vi "String functions.vi"() -> ()   [LabVIEW 2020]
panel:
  out "current time":timestamp
  out "String 6":string
  out "Boolean 2":bool
  out "Numeric 2":dbl
  out "Output Cluster":T1
  in  "String 5":string
  in  "Boolean":bool
  in  "Numeric":dbl
  out "replaced substring":string
  out "result string":string
  in  "length (len. of substring)":i32
  in  "offset (0) 2":i32
  in  "Substring":string
  in  "Main String":string
  out "substring":string
  in  "Input String":string
  in  "length (rest)":i32
  in  "offset (0)":i32
  out "concatenated string":string
  in  "String 4":string
  in  "String 3":string
  in  "String 2":string
  in  "String":string
  out "String Length":dbl
  in  "String Input":string
  # "(1)"
  # "(2)"
  # "(3)"
  # "(4)"
  # "(5)"
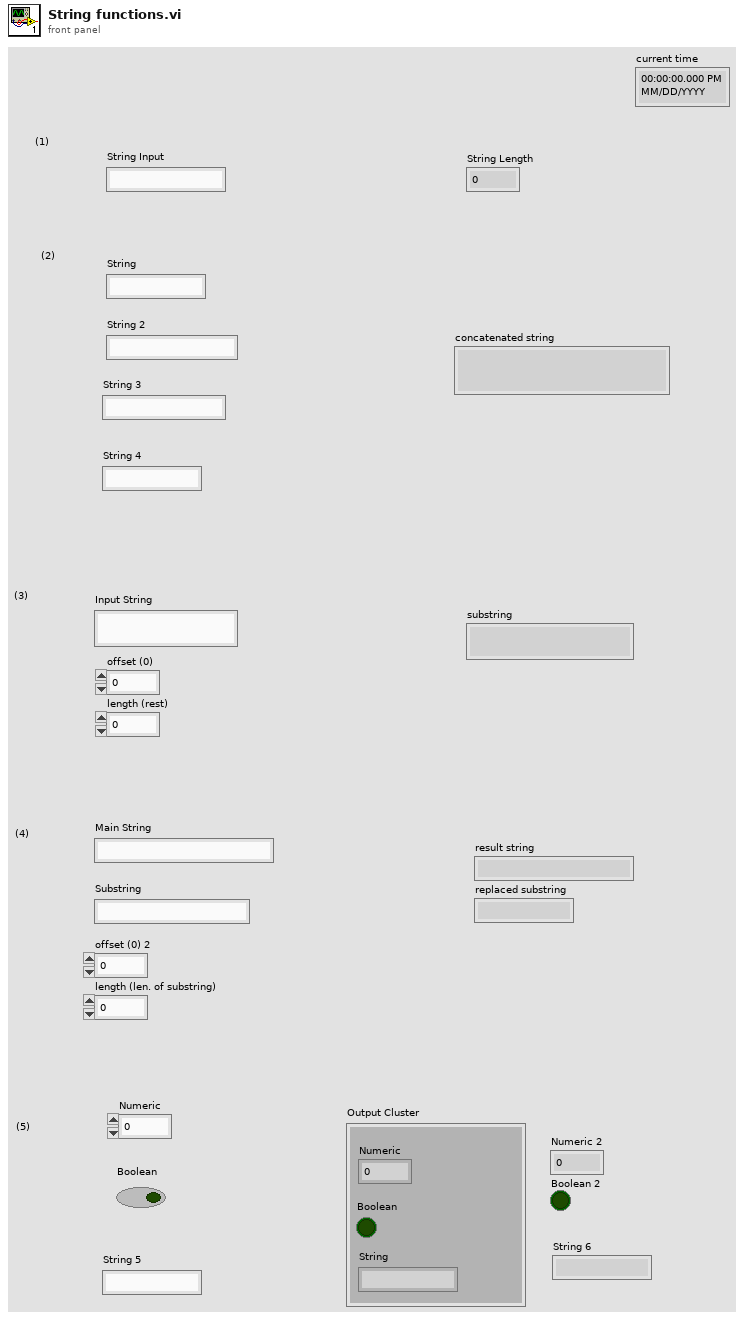
[diagram p1: front panel]
types:
  T1 = cluster{"Numeric":dbl, "Boolean":bool, "String":string}
  T2 = cluster{"Numeric":dbl, "Boolean":bool, "String 5":string}
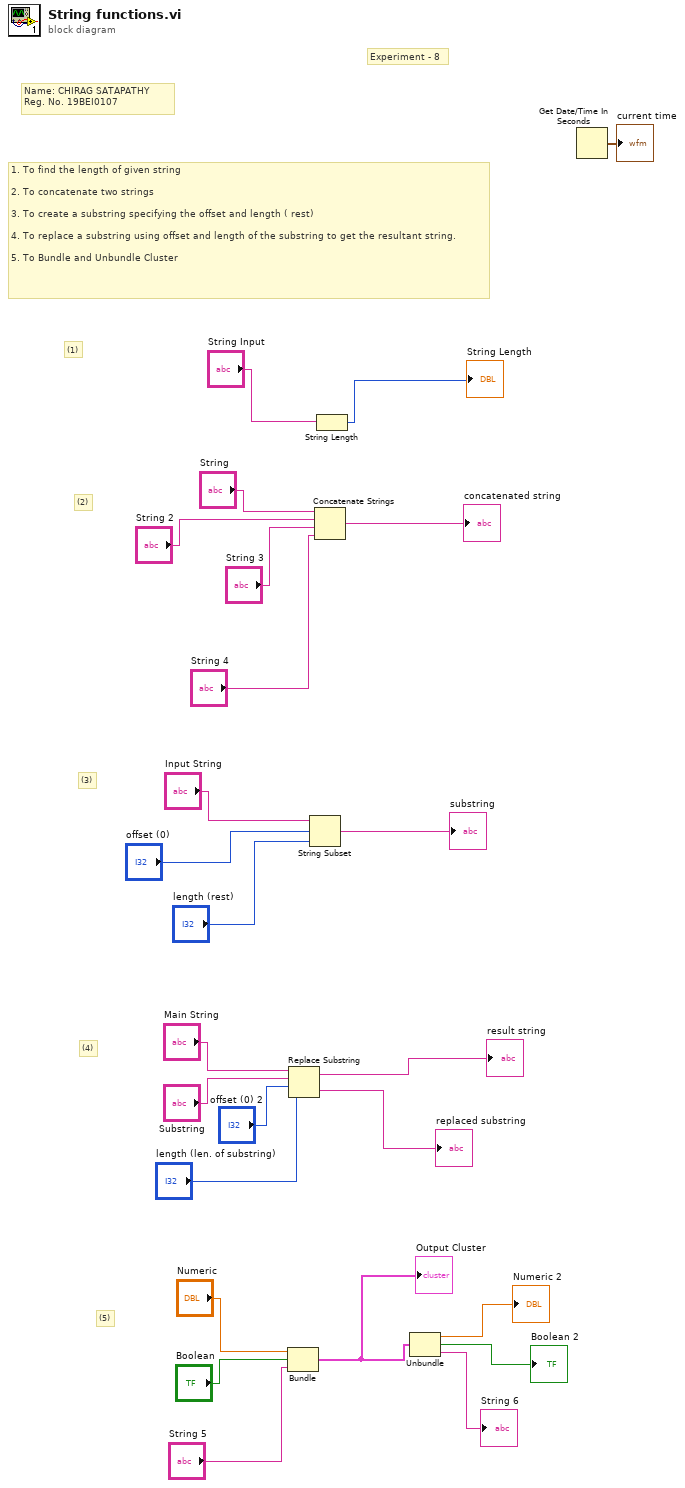
[diagram p0: block diagram]
diagram:
  # "(5)"
  # "(4)"
  # "(3)"
  # "Name: CHIRAG SATAPATHY\nReg. No. 19BEI0107"
  # "Experiment - 8"
  # "(2)"
  # "(1)"
  # "1. To find the length of given string\n\n2. To concatenate two strings\n\n3. To create a substring specifying the offset and length ( rest)\n\n4. To replace a substring using offset and length of the substring to get the resultant string.\n\n5. To Bundle and Unbundle Cluster"
  n1 = Bundle("Numeric"="Numeric", "Boolean"="Boolean", "String 5"="String 5") -> (w2:T2)  [unwired: 1 in]
  "Output Cluster" <- w2
  n2 = Replace Substring(2:"length (len. of substring)", 3:"offset (0) 2", 4:"Substring", 5:"Main String") -> (0:→"replaced substring":string, 1:→"result string":string)
  n3 = String Subset(string="Input String", offset (0)="offset (0)", length (rest)="length (rest)") -> (substring=→"substring":string)
  n4 = Concatenate Strings("String", "String 2", "String 3", "String 4") -> (→"concatenated string":string)
  n5 = String Length(string="String Input") -> (length=→"String Length":i32)
  n6 = Unbundle(w2) -> ("Numeric"=→"Numeric 2":dbl, "Boolean"=→"Boolean 2":bool, "String 5"=→"String 6":string)
  n7 = Get Date/Time In Seconds() -> (seconds since 1Jan1904=→"current time":timestamp)
